vi "Autonomous Independent.vi"() -> ()   [LabVIEW 2014]
doc: "This VI is called when autonomous begins, and will automatically be terminated when autonomous ends. You can carry out timed or sensor driven robot movement independently without needing to return to the caller."
uses:
  <vilib>/Rock Robotics/WPI/Joystick/WPI_JoystickGetSetRefNum.vi
  <vilib>/Rock Robotics/Network Tables/SD Read Numeric Array.vi
panel:
  in  "stop":bool
  # "Be sure to right-click and choose Data Operations>>Make Current Value default if you want to save the array values with the VI"
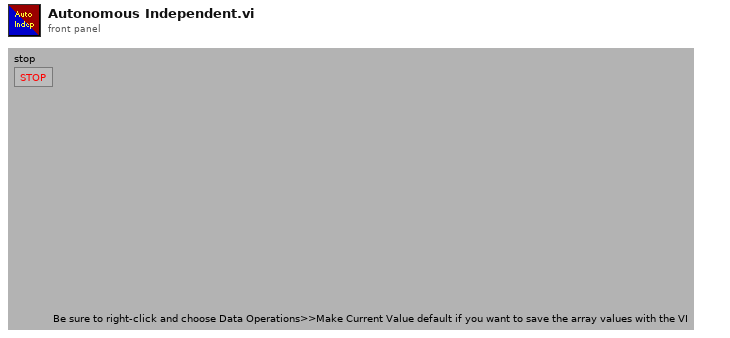
[diagram p1: front panel]
types:
  T1 = typedef "WPI_JoystickDevRef.ctl" = cluster{"Device":T2}
  T2 = typedef "WPI_JoystickDeviceEnum.ctl" = enum16{"USB 0", "USB 1", "USB 2", "USB 3", "USB 4", "USB 5"}
  T3 = cluster{"Numeric Array[0]":dbl, "Numeric Array[1]":dbl, "Numeric Array[2]":dbl, "Numeric Array[3]":dbl, "Numeric Array[4]":dbl, "Numeric Array[5]":dbl, "Numeric Array[6]":dbl, "Numeric Array[7]":dbl, "Numeric Array[8]":dbl}
  T4 = typedef "WPI_DigitalInputDevRef.ctl" = cluster{"DevStatus":errorcluster, "DIO Channel":T5, "Controller":T6}
  T5 = typedef "FPGA_DIOChannel.ctl" = enum8{"DIO 0", "DIO 1", "DIO 2", "DIO 3", "DIO 4", "DIO 5", "DIO 6", "DIO 7", "DIO 8", "DIO 9", "DIO MXP 0", "DIO MXP 1", "DIO MXP 2", "DIO MXP 3", "DIO MXP 4", "DIO MXP 5", "DIO MXP 6", "DIO MXP 7", "DIO MXP 8", "DIO MXP 9", "DIO MXP 10", "DIO MXP 11", "DIO MXP 12", "DIO MXP 13", "DIO MXP 14", "DIO MXP 15", "Invalid"}
  T6 = typedef "FPGA_TypedefDigitalModule.ctl" = enum16{"Controller 1"}
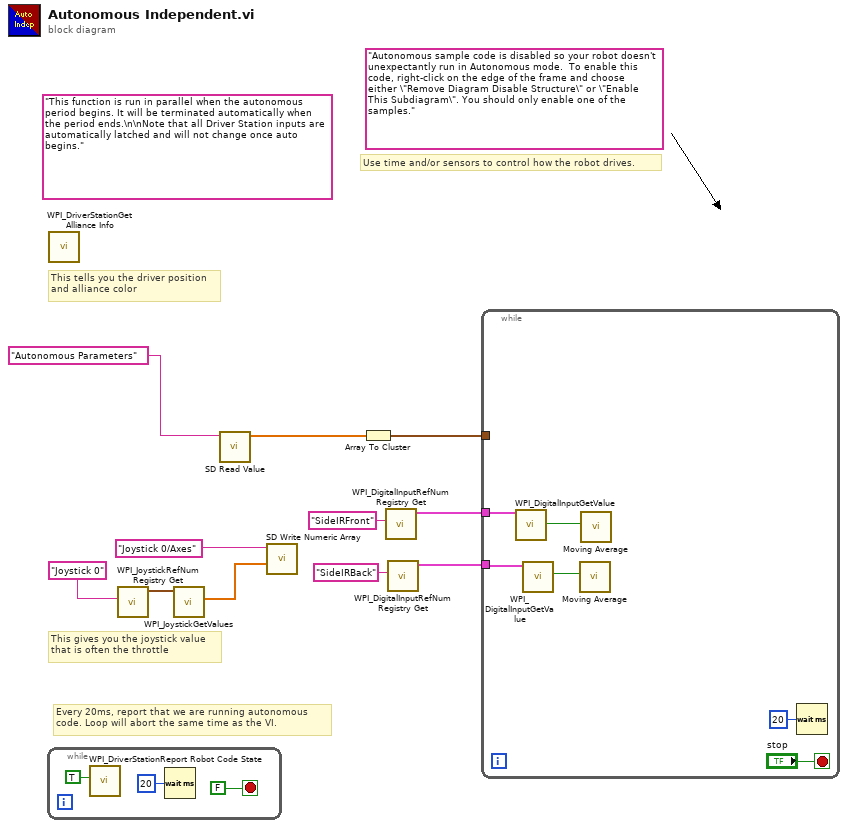
[diagram p0: block diagram]
diagram:
  (unwired) "Autonomous sample code is disabled so your robot doesn't unexpectantly run in Autonomous mode.  To enable this code, right-click on the edge of the frame and choose either \"Remove Diagram Disable Structure\" or \"Enable This Subdiagram\". You should only enable one of the samples."
  (unwired) "This function is run in parallel when the autonomous period begins. It will be terminated automatically when the period ends.\n\nNote that all Driver Station inputs are automatically latched and will not change once auto begins."
  # "Every 20ms, report that we are running autonomous\ncode. Loop will abort the same time as the VI."
  # "This gives you the joystick value\nthat is often the throttle"
  # "Use time and/or sensors to control how the robot drives."
  # "This tells you the driver position\nand alliance color"
  n1 = while {
    stop <- FALSE stop-if-true
    n2 = call <vilib>:"WPI_DriverStationReport Robot Code State.vi"("Autonomous"=TRUE) -> ()  [unwired: 10 in, 1 out]
    n3 = Wait (ms)(milliseconds to wait=u32 20) -> ()  [unwired: 1 out]
  }
  n4 = call <vilib>:"WPI_DriverStationGet Alliance Info.vi"() -> ()  [unwired: 12 out]
  n5 = call <vilib>:"WPI_JoystickRefNum Registry Get.vi"("refnum name"="Joystick 0") -> ("JoystickDevRef"=w10:T1)  [unwired: 1 in, 9 out]
  n6 = call <vilib>:"WPI_JoystickGetValues.vi"("JoystickDevRef"=w10) -> ("Axes"=w8:dbl[])  [unwired: 6 in, 4 out]
  n7 = call-poly <vilib>:"SD Read Value.vi"("Name"="Autonomous Parameters") -> ("Numeric Array"=w5:dbl[])  [unwired: 8 in, 2 out]
  n8 = call <vilib>:"SD Write Numeric Array.vi"("Numeric Array"=w8, "Name"="Joystick 0/Axes") -> ()  [unwired: 8 in, 2 out]
  n9 = Array To Cluster(array=w5) -> (cluster=w6:T3)
  n10 = call <vilib>:"WPI_DigitalInputRefNum Registry Get.vi"("refnum name"="SideIRFront") -> ("DigitalInputDevRef"=w2:T4)  [unwired: 9 in, 1 out]
  n11 = call <vilib>:"WPI_DigitalInputRefNum Registry Get.vi"("refnum name"="SideIRBack") -> ("DigitalInputDevRef"=w1:T4)  [unwired: 9 in, 1 out]
  n12 = while {
    tunnel: w6 -> [_]
    tunnel: w2 -> [w18]
    tunnel: w1 -> [w17]
    stop <- "stop" stop-if-true
    n13 = call <vilib>:"WPI_DigitalInputGetValue.vi"("DigitalInputDevRef"=w18) -> ("Value"=w16:bool)  [unwired: 8 in, 2 out]
    n14 = call <vilib>:"WPI_DigitalInputGetValue.vi"("DigitalInputDevRef"=w17) -> ("Value"=w15:bool)  [unwired: 8 in, 2 out]
    n15 = call "Moving Average.vi"("Value"=w15) -> ()  [unwired: 10 in, 1 out]
    n16 = call "Moving Average.vi"("Value"=w16) -> ()  [unwired: 10 in, 1 out]
    n17 = Wait (ms)(milliseconds to wait=u32 20) -> ()  [unwired: 1 out]
  }
